vi "Read Partial.vi"(11 "Series in":refnum<class "Series.lvclass">) -> (2 "Partial":bool, 3 "Series out":refnum<class "Series.lvclass">)   [LabVIEW 2018, in "InfluxDB Client.lvlib" / "Series.lvclass"]
uses:
  Series.lvclass
  Series.lvclass/Series.ctl
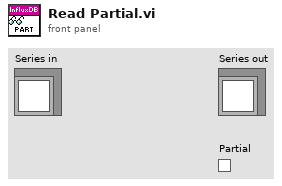
[diagram p1: front panel]
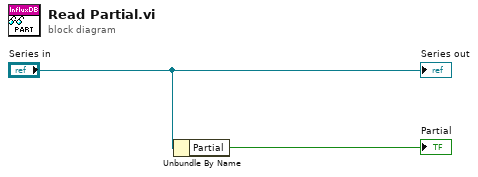
[diagram p0: block diagram]
diagram:
  n1 = Unbundle By Name("Series in") -> ("Partial"=→"Partial":bool)
  "Series out" <- "Series in"
